vi "Backward SubVi.vi"(10 "Numeric":i32, 11 "Array":cluster{"Horizontal":i32, i32}[](array[cluster])) -> (2 "Cluster 2":cluster{"Horizontal":dbl, dbl}, 3 "Cluster":cluster{"Horizontal":i32, i32})   [LabVIEW 2014]
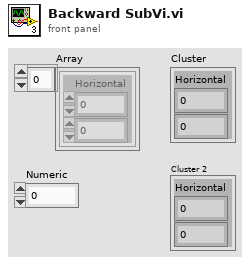
[diagram p1: front panel]
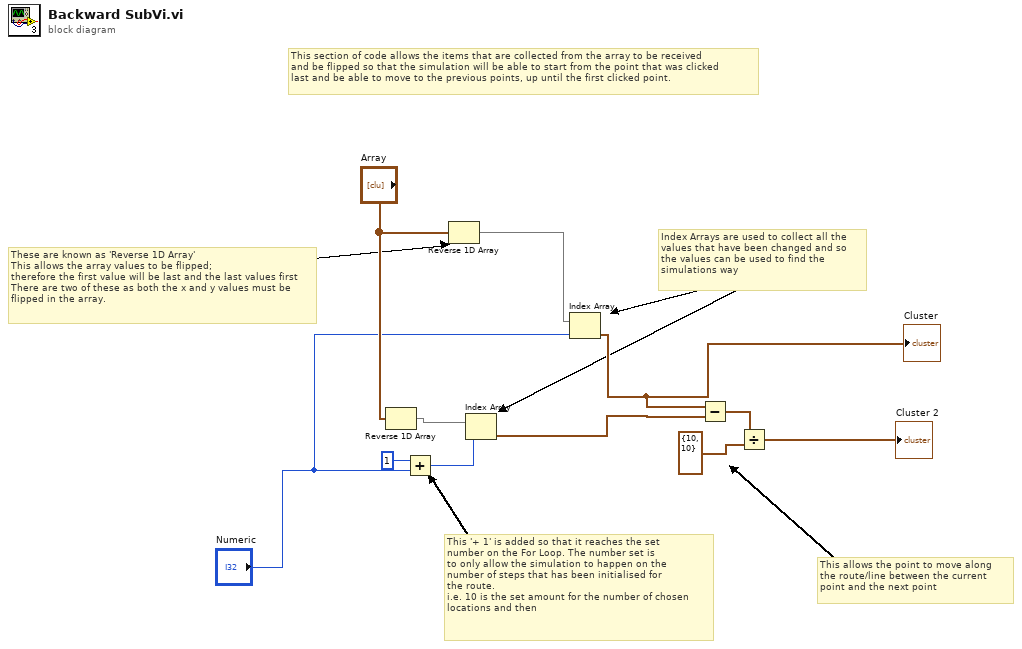
[diagram p0: block diagram]
diagram:
  # "Index Arrays are used to collect all the\nvalues that have been changed and so \nthe values can be used to find the \nsimulations way"
  # "This allows the point to move along \nthe route/line between the current\npoint and the next point"
  # "This '+ 1' is added so that it reaches the set\nnumber on the For Loop. The number set is \nto only allow the simulation to happen on the\nnumber of steps that has been initialised for \nthe route. \ni.e. 10 is the set amount for the number of chosen \nlocations and then"
  # "These are known as 'Reverse 1D Array' \nThis allows the array values to be flipped; \ntherefore the first value will be last and the last values first\nThere are two of these as both the x and y values must be \nflipped in the array."
  # "This section of code allows the items that are collected from the array to be received\nand be flipped so that the simulation will be able to start from the point that was clicked \nlast and be able to move to the previous points, up until the first clicked point."
  n1 = Reverse 1D Array(array="Array") -> (reversed array=w2:cluster{"Horizontal":i32, i32}[])
  n2 = Add(x=1, y="Numeric") -> (x+y=w8:i32)
  n3 = Reverse 1D Array(array="Array") -> (reversed array=w11:cluster{"Horizontal":i32, i32}[])
  n4 = Index Array(array=w2, index=w8) -> (element=w6:cluster{"Horizontal":i32, i32})
  n5 = Index Array(array=w11, index="Numeric") -> (element=w7:cluster{"Horizontal":i32, i32})
  "Cluster" <- w7
  n6 = Subtract(x=w7, y=w6) -> (x-y=w3:cluster{"Horizontal":i32, i32})
  n7 = Divide(x=w3, y=cluster{"Horizontal":i32, i32} {"Horizontal"=10, 10}) -> (x/y=→"Cluster 2":cluster{"Horizontal":dbl, dbl})
